vi "roundBuoy.vi"(11 "RoundBuoys in":refnum<class "RoundBuoy.lvclass">) -> (3 "RoundBuoys out":refnum<class "RoundBuoy.lvclass">)   [LabVIEW 2011, in "RoundBuoy.lvclass"]
doc: "ROUND BUOY VI\n\nThis VI enables the boat to drive around a buoy in either CW or CCW direction.\nThe UTM coordinates, the rounding direction and a variable for distance tolerance create two points around the buoy.\nThose poins will be defined as start and endpoint of the rounding.\nA third point, which defines the way around the buoy has to be set now.\nA line with 5 possible waypoints is created in an fixed angle from the endpoint towards the starting point.\nDepending on the wind direction, the point which allows the fastest boat speed towards this point is chosen as wypoint.\nThise Points are then inserted into the waypoint array."
uses:
  RoundBuoy.lvclass
  2 Typedefs/UTM Location.ctl
  2 Typedefs/Velocity.ctl
  RoundBuoy.lvclass/RoundBuoy.ctl
  GenericMission/GenericMission.lvclass
  2 Globals/2 Global.vi
  Waypoint/Waypoint.lvclass
  MissionQueue/MissionQueue.lvclass
panel:
  out "Exit Waypoint":T1 {"North" format="%#_10f"; "East" format="%#_8f"}
  out "Entry Waypoint":T1 {"North" format="%#_10f"; "East" format="%#_8f"}
  out "Second Waypoint":T1 {"North" format="%#_10f"; "East" format="%#_8f"}
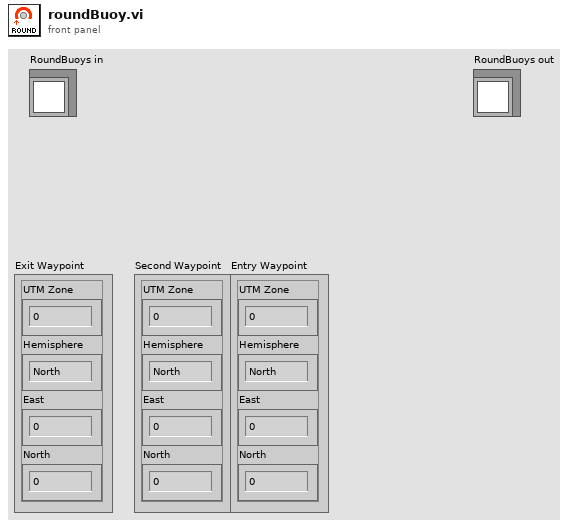
[diagram p1: front panel]
types:
  T1 = typedef "UTM Location.ctl" = cluster{"UTM Zone":dbl, "Hemisphere":enum16{"North", "South"}, "East":dbl, "North":dbl}
  T2 = typedef "Velocity.ctl" = cluster{"East":dbl, "North":dbl}
  T3 = cluster{"UTM Zone":dbl, "Hemisphere":u16, "East":dbl, "North":dbl}
  T4 = typedef "heading.ctl" = dbl
  T5 = typedef "Waypoints List.ctl" = refnum<class "Waypoint.lvclass">[]
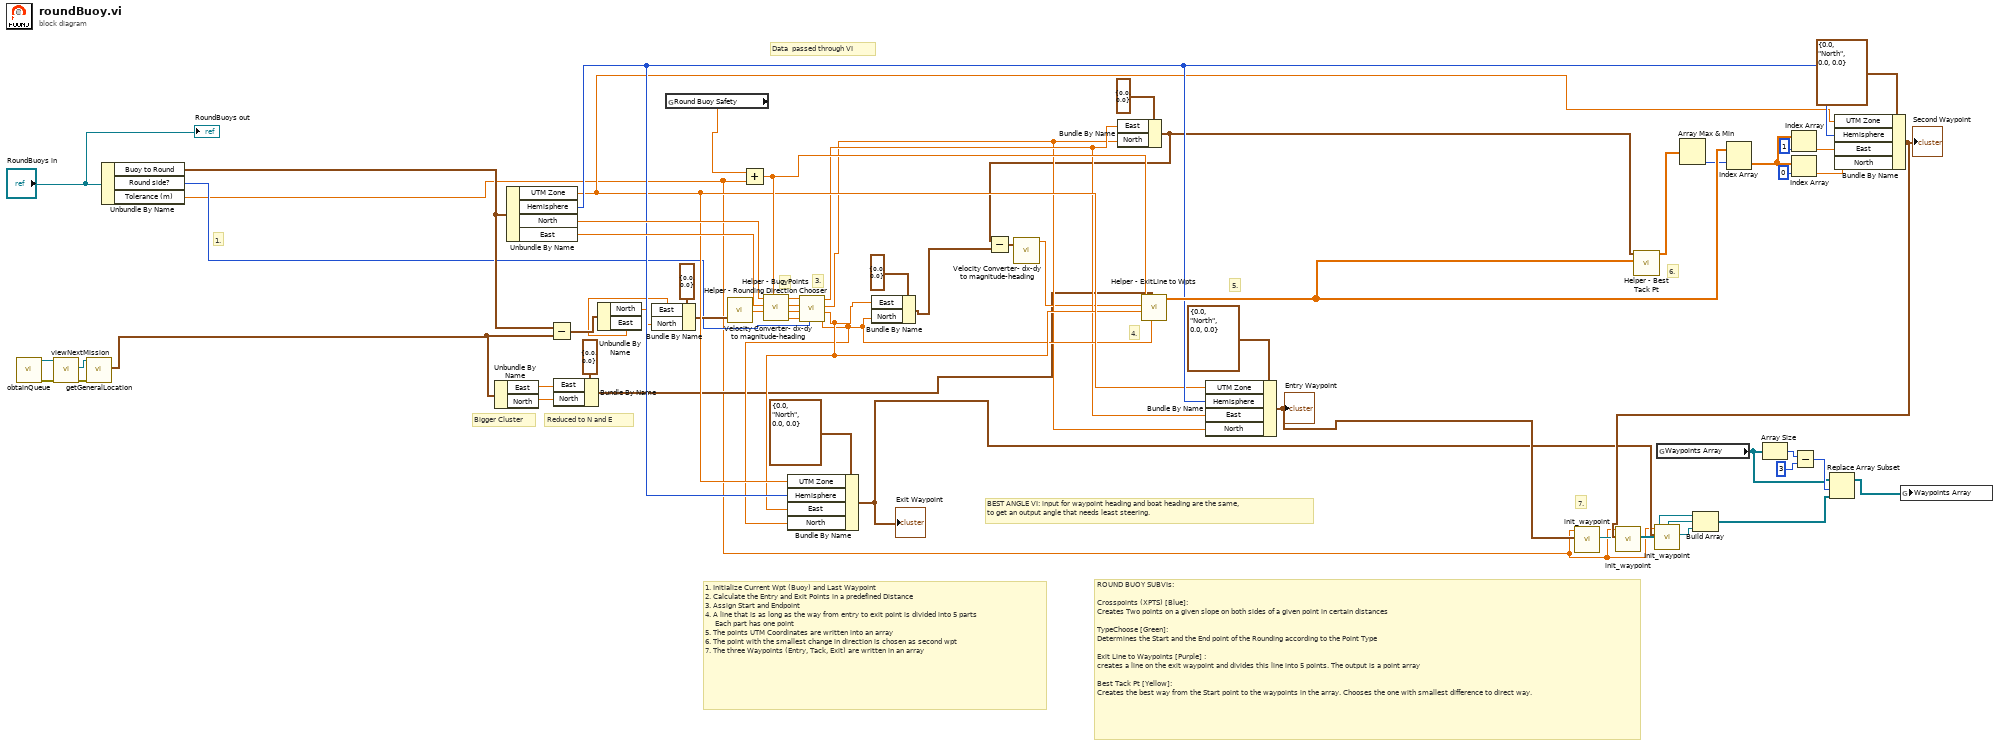
[diagram p0: block diagram]
diagram:
  # "3."
  # "ROUND BUOY SUBVIs:\n\nCrosspoints (XPTS) [Blue]:\nCreates Two points on a given slope on both sides of a given point in certain distances\n\nTypeChoose [Green]:\nDetermines the Start and the End point of the Rounding according to the Point Type\n\nExit Line to Waypoints [Purple] :\ncreates a line on the exit waypoint and divides this line into 5 points. The output is a point array\n\nBest Tack Pt [Yellow]:\nCreates the best way from the Start point to the waypoints in the array. Chooses the one with smallest difference to direct way."
  # "BEST ANGLE VI: input for waypoint heading and boat heading are the same,\nto get an output angle that needs least steering."
  # "Reduced to N and E"
  # "Bigger Cluster"
  # "Data  passed through VI"
  # "7."
  # "6."
  # "5."
  # "1. Initialize Current Wpt (Buoy) and Last Waypoint\n2. Calculate the Entry and Exit Points in a predefined Distance\n3. Assign Start and Endpoint\n4. A line that is as long as the way from entry to exit point is divided into 5 parts\n     Each part has one point\n5. The points UTM Coordinates are written into an array\n6. The point with the smallest change in direction is chosen as second wpt\n7. The three Waypoints (Entry, Tack, Exit) are written in an array"
  # "4."
  # "2."
  # "1."
  n1 = call "obtainQueue.vi"() -> ("Error Out"=w6:errorcluster, "MissionQueue.lvclass"=w5:refnum<class "MissionQueue.lvclass">)  [unwired: 10 in]
  n2 = call "viewNextMission.vi"("error in (no error)"=w6, "MissionQueue in"=w5) -> ("error out"=w4:errorcluster, "GenericMission.lvclass"=w3:refnum<class "GenericMission.lvclass">)  [unwired: 6 in, 2 out]
  n3 = call-dynamic "getGeneralLocation.vi"("error in (no error)"=w4, "GenericMission in"=w3) -> ("General Location"=w2:T1)  [unwired: 7 in, 2 out]
  n4 = Unbundle By Name("RoundBuoys in") -> ("Buoy to Round"=w10:T1, "Round side?"=w9:enum16{"Starboard", "Port"}, "Tolerance (m)"=w8:dbl)
  n5 = Unbundle By Name(w2) -> ("East"=w60:dbl, "North"=w59:dbl)
  n6 = Unbundle By Name(w10) -> ("UTM Zone"=w42:dbl, "Hemisphere"=w43:enum16{"North", "South"}, "North"=w62:dbl, "East"=w61:dbl)
  n7 = Subtract(x=w10, y=w2) -> (x-y=w37:T3)
  n8 = Bundle By Name(cluster=T2 {"East"=0.0, "North"=0.0} ("Vector In"), "East"=w60, "North"=w59) -> (w11:T2)
  n9 = Unbundle By Name(w37) -> ("North"=w35:dbl, "East"=w32:dbl)
  n10 = Bundle By Name(cluster=T2 {"East"=0.0, "North"=0.0} ("Vector In"), "East"=w32, "North"=w35) -> (w34:T2)
  n11 = global read "2 Global.vi" "Round Buoy Safety"() -> (w1:dbl)
  n12 = call "Velocity Converter- dx-dy to magnitude-heading.vi"("Vector In"=w34) -> ("Heading Out"=w33:T4)  [unwired: 9 in, 1 out]
  n13 = Add(x=w1, y=w8) -> (x+y=w56:dbl)
  n14 = call "Helper - BuoyPoints.vi"("Distance"=w56, "K"=w33, "East"=w61, "North"=w62) -> ("NorthOut 2"=w38:dbl, "East Out 2"=w39:dbl, "NorthOut"=w40:dbl, "East Out"=w41:dbl)  [unwired: 4 in]
  n15 = call "Helper - Rounding Direction Chooser.vi"("Buoy\nSide"=w9, "Point NORTH 2"=w38, "Point EAST 2"=w39, "Point NORTH"=w40, "Point EAST"=w41) -> ("End Point NORTH"=w20:dbl, "End Point EAST"=w21:dbl, "Start Point NORTH"=w18:dbl, "Start Point EAST"=w19:dbl)  [unwired: 3 in]
  n16 = Bundle By Name(cluster=T1 {"UTM Zone"=0.0, "Hemisphere"=enum."North", "East"=0.0, "North"=0.0} ("UTM Location"), "UTM Zone"=w42, "Hemisphere"=w43, "East"=w21, "North"=w20) -> (w16:T1)
  "Exit Waypoint" <- w16
  n17 = Bundle By Name(cluster=T2 {"East"=0.0, "North"=0.0} ("Vector In"), "East"=w21, "North"=w20) -> (w14:T2)
  n18 = Bundle By Name(cluster=T2 {"East"=0.0, "North"=0.0} ("Vector In"), "East"=w19, "North"=w18) -> (w15:T2)
  n19 = Subtract(x=w15, y=w14) -> (x-y=w13:T2)
  n20 = call "Velocity Converter- dx-dy to magnitude-heading.vi"("Vector In"=w13) -> ("Heading Out"=w12:T4)  [unwired: 9 in, 1 out]
  n21 = call "Helper - ExitLine to Wpts.vi"("North In"=w20, "Next Point"=w11, "East In"=w21, "Best Angle"=w12, "Distance"=w56) -> ("Point on Line"=w53:dbl[][])  [unwired: 6 in]
  n22 = Bundle By Name(cluster=T1 {"UTM Zone"=0.0, "Hemisphere"=enum."North", "East"=0.0, "North"=0.0} ("UTM Location"), "UTM Zone"=w42, "Hemisphere"=w43, "East"=w19, "North"=w18) -> (w17:T1)
  "Entry Waypoint" <- w17
  n23 = call "init_waypoint.vi"("Coords"=w17, "Tolerance (m)"=w8) -> ("Waypoint Out"=w29:refnum<class "Waypoint.lvclass">)  [unwired: 9 in]
  n24 = call "Helper - Best Tack Pt.vi"("Point on Line"=w53, "Vector In"=w15) -> ("Array"=w54:dbl[])  [unwired: 9 in]
  n25 = call "init_waypoint.vi"("Coords"=w16, "Tolerance (m)"=w8) -> ("Waypoint Out"=w27:refnum<class "Waypoint.lvclass">)  [unwired: 9 in]
  n26 = global read "2 Global.vi" "Waypoints Array"() -> (w24:T5)
  n27 = Array Max & Min(array=w54) -> (min index (indices)=w52:i32)  [unwired: 3 out]
  n28 = Index Array(array=w53, index (row)=w52) -> (element=w47:dbl[])  [unwired: 1 in]
  n29 = Array Size(array=w24) -> (size(s)=w30:i32)
  n30 = Index Array(array=w47, index=1) -> (element=w49:dbl)
  n31 = Index Array(array=w47, index=0) -> (element=w48:dbl)
  n32 = Subtract(x=w30, y=3) -> (x-y=w25:i32)
  n33 = Bundle By Name(cluster=T1 {"UTM Zone"=0.0, "Hemisphere"=enum."North", "East"=0.0, "North"=0.0} ("UTM Location"), "UTM Zone"=w42, "Hemisphere"=w43, "East"=w49, "North"=w48) -> (w31:T1)
  "Second Waypoint" <- w31
  n34 = call "init_waypoint.vi"("Coords"=w31, "Tolerance (m)"=w8) -> ("Waypoint Out"=w28:refnum<class "Waypoint.lvclass">)  [unwired: 9 in]
  n35 = Build Array(w29, w28, w27) -> (w23:refnum<class "Waypoint.lvclass">[])
  n36 = Replace Array Subset(array=w24, new element=w23, index=w25) -> (w22:T5)
  n37 = global write "2 Global.vi" "Waypoints Array"(w22) -> ()
  "RoundBuoys out" <- "RoundBuoys in"
